vi "TestLV_RT Driver VI.vi"(6 "Device Clock":string) -> ()   [LabVIEW 2017]
uses:
  Par.ctl
  LambdaType.ctl
  Sensor_used.ctl
  <vilib>/Platform/TimedLoop/XDataNode/timing_clust.ctl
  <vilib>/Platform/TimedLoop/XDataNode/nitl_modes.ctl
  <vilib>/Platform/TimedLoop/XDataNode/wakeup.ctl
  <vilib>/SLSC/Initialize Session with Devices.vi
  <vilib>/SLSC/Close Session.vi
  <vilib>/Platform/TimedLoop/XDataNode/XDataNode.xnode
  <vilib>/Platform/TimedLoop/XDataNode/XDNodeRunTimeDep.lvlib
  ALMA_10201-10401_O2SensorSim Engine.lvlib
  <vilib>/SLSC/SLSC.lvlib
  <resource>/objmgr/slsc.rc
panel:
  in  "Feedback 3":string[](array[string])=["Lambda Feedback", "Status", "Duty Cycle Heater", "Frequency Heater", "Ip", "Ri", "V_Ip", "V_Ri"]
  in  "Feedback 2":string[](array[string])=["Lambda Feedback", "Status", "Duty Cycle Heater", "Frequency Heater", "Ip", "Ri", "V_Ip", "V_Ri"]
  in  "Feedback":string[](array[string])=["Lambda Feedback", "Status", "Duty Cycle Heater", "Frequency Heater", "Ip", "Ri", "V_Ip", "V_Ri"]
  in  "Setpoint 2":string[](array[string])=["Enable_1", "Lambda Target_1", "Sensor Temp_1", "Enable_3", "Lambda Target_3", "Sensor Temp_3"]
  in  "Setpoint":string[](array[string])=["Enable_1", "Lambda Target_1", "Sensor Temp_1", "Enable_2", "Lambda Target_2", "Sensor Temp_2", "Enable_3", "Lambda Target_3", "Sensor Temp_3", "Enable_4", "Lambda Target_4", "Sensor Temp_4"]
  in  "Array":T1[](array[typedef])=[0, 1, 2, 3] items=["LSU4.2", "LSU4.9", "LZA03", "LZA08", "Custom", "[mA]"]
  in  "Tab Control":enum32{"Page 1", "Page 2", "Page 3", "Page 4"}(tab)
  out "Temperature [°C] VS Rs [W]":cluster{"Custom Temp":dbl[], "Custom Ohm":dbl[]}(graph)
  out "l VS IP [mA]":T2(graph)
  in  "Mode":enum16{"SLSC Mode", "ANALOG Mode"}(ring)
  out "decimal integer string":string
  out "Dev.ProductName":string
  out "Dev.VendorNum":u32
  out "Dev.ProductNum":u32
  out "output cluster":T3
  out "VS feedback 2":dbl[](array[numeric])=[1.0032000541687012, 0.0, 0.0, 0.0, 1.0032000541687012, 0.0, 99.0, 0.0, -2.0, 1000.0, -2.0, 1000.0, 0.0, 0.0, 3.333400011062622, 9.309800148010254, 3.333400011062622, 9.309800148010254]
  in  "VS control 2":dbl[](array[numeric])=[0.0, 0.0, 0.0, 0.0, 0.0, 0.0, 0.0, 0.0, 0.0, 0.0, 0.0, 0.0, 0.0, 0.0, 0.0]
  in  "#ch_choise":enum16{"O2Sim_2ch", "O2Sim_4ch"}(ring)
  in  "SensorUsed 2":T3
  in  "Next_IP 1":u32=192 caption="O2SensorSim IP"
  in  "Next_IP 4":u32=4
  in  "Next_IP 2":u32=168
  in  "Next_IP 3":u32=1
  out "error out 2":errorcluster
  out "error out":errorcluster
  out "VS feedback":dbl[](array[numeric])
  in  "stop":bool
  in  "VS control":dbl[](array[numeric])=[0.0, 0.0, 0.0, 0.0, 0.0, 0.0, 0.0, 0.0, 0.0, 0.0, 0.0, 0.0, 0.0, 0.0, 0.0, 0.0, 0.0, 0.0, 0.0, 0.0, 0.0]
  in  "devices":refnum<k21>="SLSC-12001-0310EC4F-Mod1"
  in  "par":T4={"Loop time"={"Loop Rate"=0, "Processor"=0}, "COM"={"COM IP"="0.0.0.0", "COM port"=1, "Local port"=0, "Next_IP 1"=0, "Next_IP 2"=0, "Next_IP 3"=0, "Next_IP 4"=0}, "O2Sensor1"={"Lambda"={"LSU4.2 Lambda"=[], "LSU4.2 Ip"=[], "LSU4.9 Lambda"=[], "LSU4.9 Ip"=[], "LZA03 Lambda"=[], "LZA03 Ip"=[], "LZA08 Lambda"=[], "LZA08 Ip"=[], "Custom Lambda"=[], "Custom Ip"=[]}, "Temp"={"LSU4.2 Temp"=[], "LSU4.2 Ohm"=[], "LSU4.9 Temp"=[], "LSU4.9 Ohm"=[], "LZA03 Temp"=[], "LZA03 Ohm"=[], "LZA08 Temp"=[], "LZA08 Ohm"=[], "Custom Temp"=[], "Custom Ohm"=[]}, "Lambda Type"=0, "PID"={"Ki"=0.0, "Kp"=0.0, "Kd"=0.0, "FeedFW"=0.0}}, "O2Sensor2"={"Lambda"={"LSU4.2 Lambda"=[], "LSU4.2 Ip"=[], "LSU4.9 Lambda"=[], "LSU4.9 Ip"=[], "LZA03 Lambda"=[], "LZA03 Ip"=[], "LZA08 Lambda"=[], "LZA08 Ip"=[], "Custom Lambda"=[], "Custom Ip"=[]}, "Temp"={"LSU4.2 Temp"=[], "LSU4.2 Ohm"=[], "LSU4.9 Temp"=[], "LSU4.9 Ohm"=[], "LZA03 Temp"=[], "LZA03 Ohm"=[], "LZA08 Temp"=[], "LZA08 Ohm"=[], "Custom Temp"=[], "Custom Ohm"=[]}, "Lambda Type"=0, "PID"={"Ki"=0.0, "Kp"=0.0, "Kd"=0.0, "FeedFW"=0.0}}, "O2Sensor3"={"Lambda"={"LSU4.2 Lambda"=[], "LSU4.2 Ip"=[], "LSU4.9 Lambda"=[], "LSU4.9 Ip"=[], "LZA03 Lambda"=[], "LZA03 Ip"=[], "LZA08 Lambda"=[], "LZA08 Ip"=[], "Custom Lambda"=[], "Custom Ip"=[]}, "Temp"={"LSU4.2 Temp"=[], "LSU4.2 Ohm"=[], "LSU4.9 Temp"=[], "LSU4.9 Ohm"=[], "LZA03 Temp"=[], "LZA03 Ohm"=[], "LZA08 Temp"=[], "LZA08 Ohm"=[], "Custom Temp"=[], "Custom Ohm"=[]}, "Lambda Type"=0, "PID"={"Ki"=0.0, "Kp"=0.0, "Kd"=0.0, "FeedFW"=0.0}}, "O2Sensor4"={"Lambda"={"LSU4.2 Lambda"=[], "LSU4.2 Ip"=[], "LSU4.9 Lambda"=[], "LSU4.9 Ip"=[], "LZA03 Lambda"=[], "LZA03 Ip"=[], "LZA08 Lambda"=[], "LZA08 Ip"=[], "Custom Lambda"=[], "Custom Ip"=[]}, "Temp"={"LSU4.2 Temp"=[], "LSU4.2 Ohm"=[], "LSU4.9 Temp"=[], "LSU4.9 Ohm"=[], "LZA03 Temp"=[], "LZA03 Ohm"=[], "LZA08 Temp"=[], "LZA08 Ohm"=[], "Custom Temp"=[], "Custom Ohm"=[]}, "Lambda Type"=0, "PID"={"Ki"=0.0, "Kp"=0.0, "Kd"=0.0, "FeedFW"=0.0}}, "Board"=0, "Mode"=enum."SLSC Mode", "vendor.Num"=4141, "product.Num"=0} {"Board" items=["O2Sim_2ch", "O2Sim_4ch"]; "O2Sensor4"."Lambda Type" items=["LSU4.2", "LSU4.9", "LZA03", "LZA08", "Custom", "[mA]"]; "O2Sensor3"."Lambda Type" items=["LSU4.2", "LSU4.9", "LZA03", "LZA08", "Custom", "[mA]"]; "O2Sensor2"."Lambda Type" items=["LSU4.2", "LSU4.9", "LZA03", "LZA08", "Custom", "[mA]"]; "O2Sensor1"."Lambda Type" items=["LSU4.2", "LSU4.9", "LZA03", "LZA08", "Custom", "[mA]"]}
  out "Device Session":refnum<k21>
  out "COM error":bool
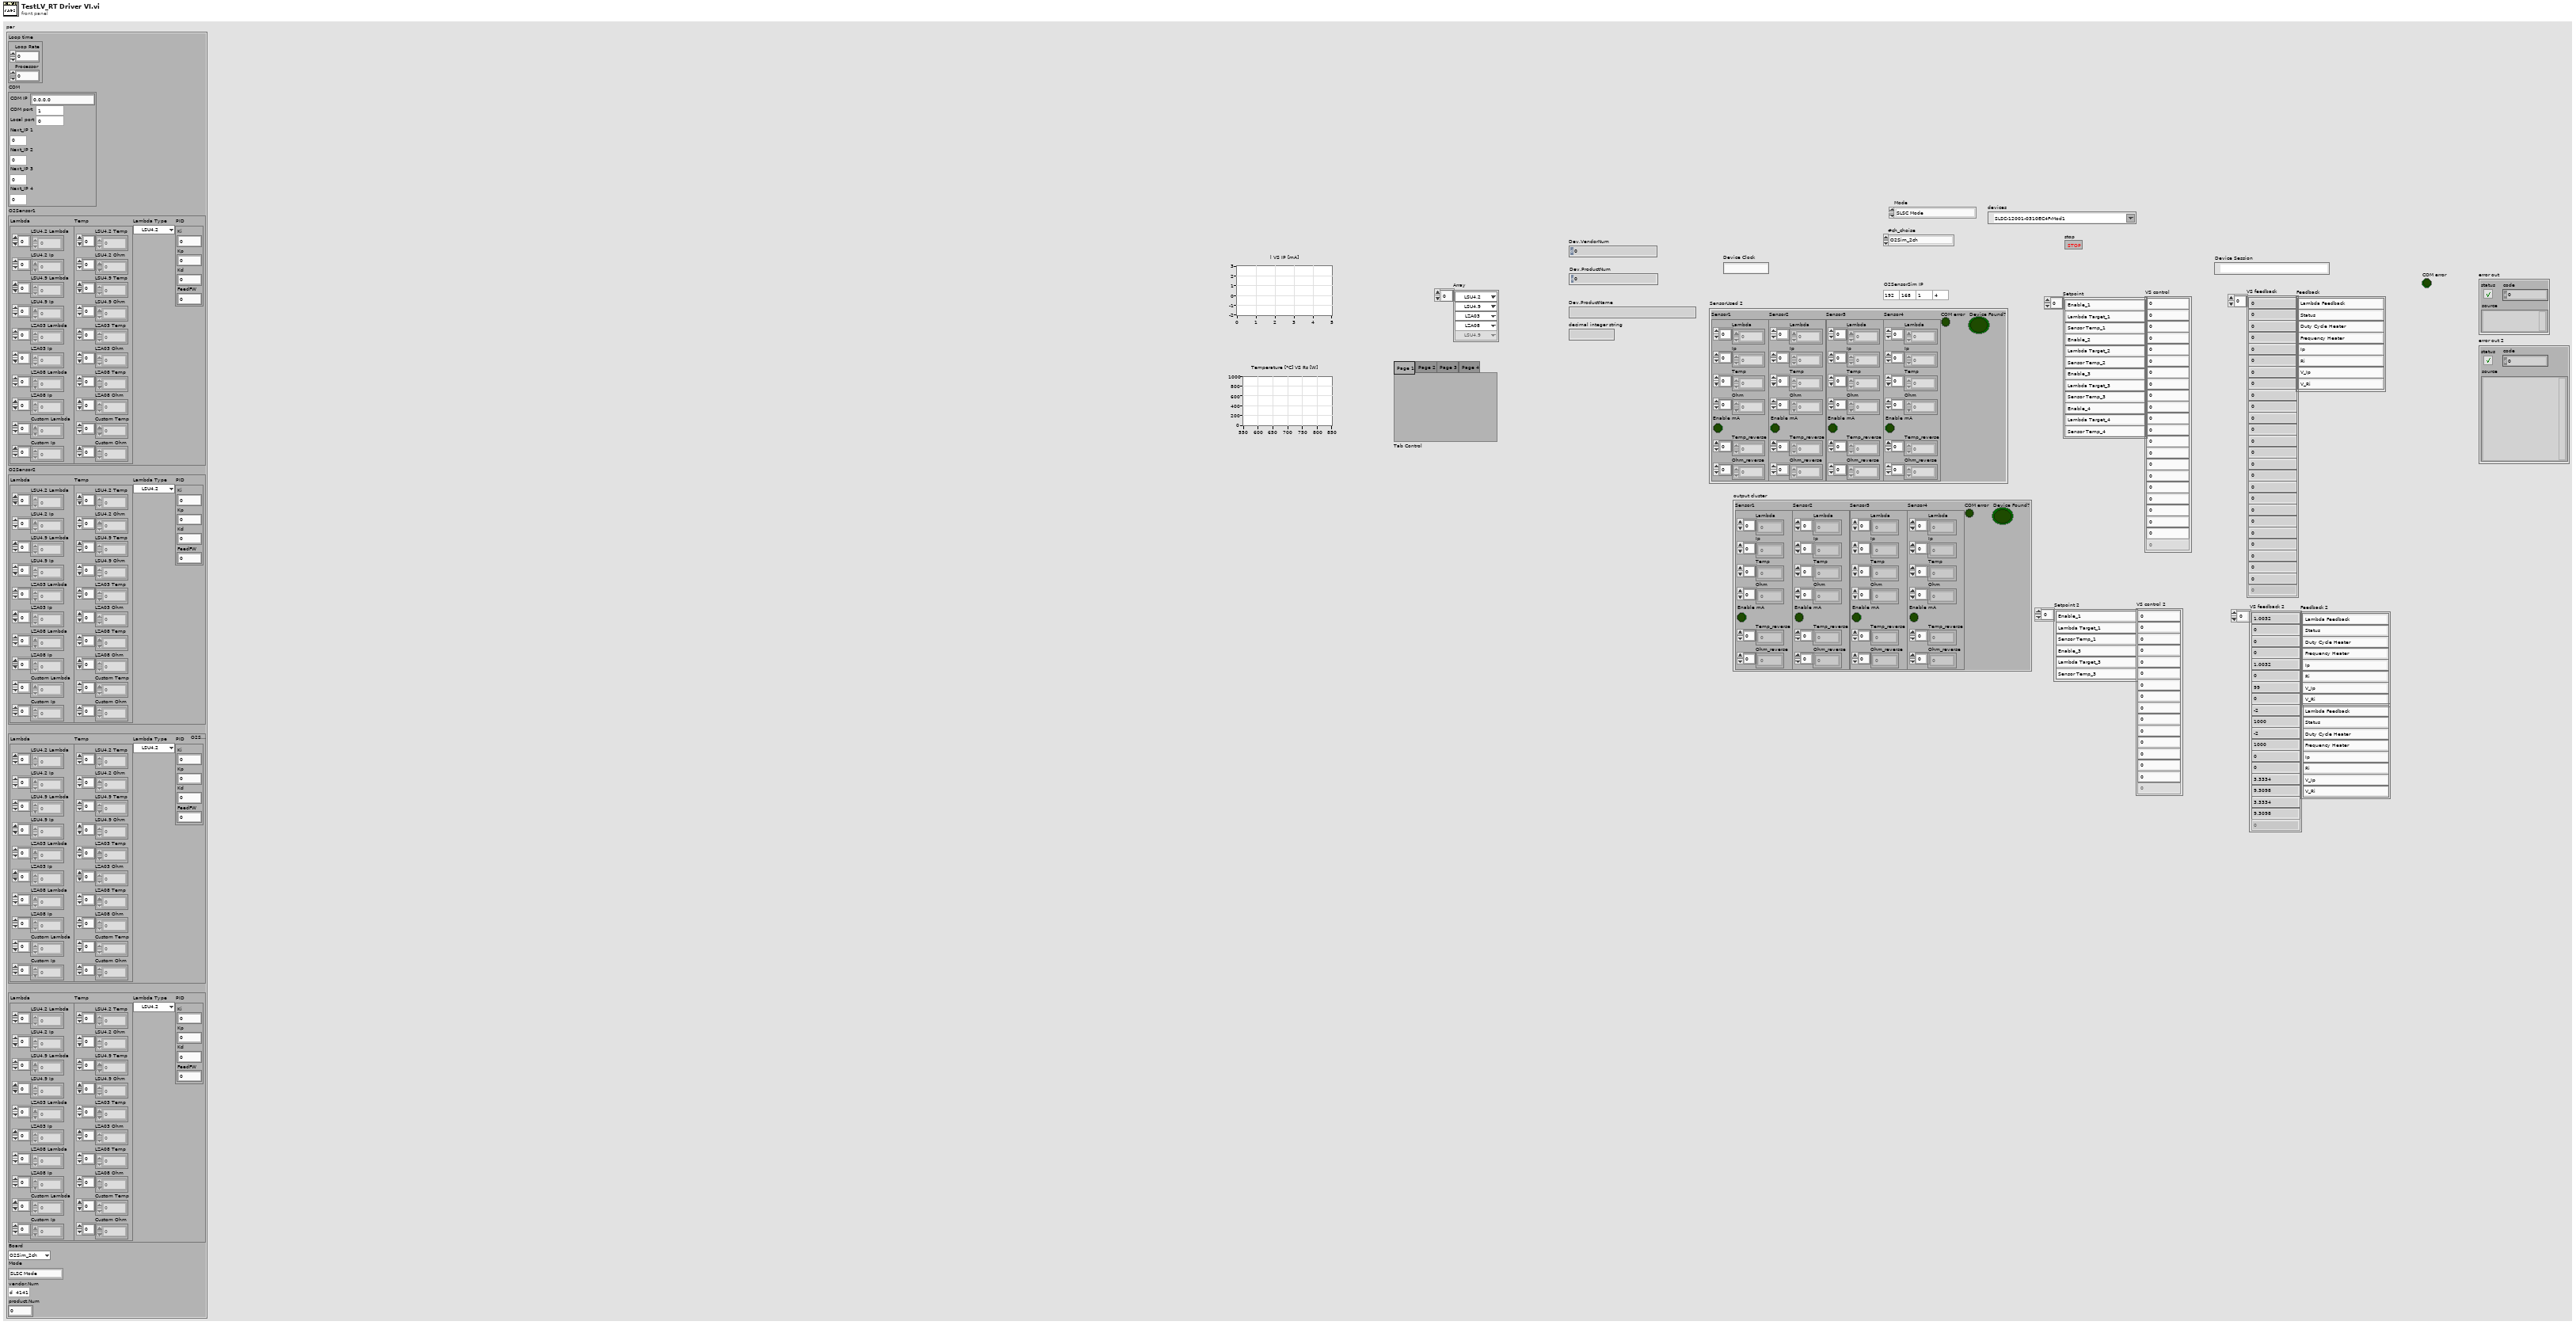
[diagram p1: front panel]
types:
  T1 = typedef "LambdaType.ctl" = u16
  T2 = cluster{"Custom Lambda":dbl[], "Custom Ip":dbl[]}
  T3 = typedef "ALMA_10201-10401_O2SensorSim Engine.lvlib/Sensor_used.ctl" = cluster{"Sensor1":cluster{"Lambda":dbl[], "Ip":dbl[], "Temp":dbl[], "Ohm":dbl[], "Enable mA":bool, "Temp_reverse":dbl[], "Ohm_reverse":dbl[]}, "Sensor2":cluster{"Lambda":dbl[], "Ip":dbl[], "Temp":dbl[], "Ohm":dbl[], "Enable mA":bool, "Temp_reverse":dbl[], "Ohm_reverse":dbl[]}, "Sensor3":cluster{"Lambda":dbl[], "Ip":dbl[], "Temp":dbl[], "Ohm":dbl[], "Enable mA":bool, "Temp_reverse":dbl[], "Ohm_reverse":dbl[]}, "Sensor4":cluster{"Lambda":dbl[], "Ip":dbl[], "Temp":dbl[], "Ohm":dbl[], "Enable mA":bool, "Temp_reverse":dbl[], "Ohm_reverse":dbl[]}, "COM error":bool, "Device Found?":bool}
  T4 = typedef "Par.ctl" = cluster{"Loop time":cluster{"Loop Rate":i64, "Processor":i32}, "COM":cluster{"COM IP":string, "COM port":u64, "Local port":u64, "Next_IP 1":u32, "Next_IP 2":u32, "Next_IP 3":u32, "Next_IP 4":u32}, "O2Sensor1":cluster{"Lambda":cluster{"LSU4.2 Lambda":dbl[], "LSU4.2 Ip":dbl[], "LSU4.9 Lambda":dbl[], "LSU4.9 Ip":dbl[], "LZA03 Lambda":dbl[], "LZA03 Ip":dbl[], "LZA08 Lambda":dbl[], "LZA08 Ip":dbl[], "Custom Lambda":dbl[], "Custom Ip":dbl[]}, "Temp":cluster{"LSU4.2 Temp":dbl[], "LSU4.2 Ohm":dbl[], "LSU4.9 Temp":dbl[], "LSU4.9 Ohm":dbl[], "LZA03 Temp":dbl[], "LZA03 Ohm":dbl[], "LZA08 Temp":dbl[], "LZA08 Ohm":dbl[], "Custom Temp":dbl[], "Custom Ohm":dbl[]}, "Lambda Type":T1, "PID":cluster{"Ki":dbl, "Kp":dbl, "Kd":dbl, "FeedFW":dbl}}, "O2Sensor2":cluster{"Lambda":cluster{"LSU4.2 Lambda":dbl[], "LSU4.2 Ip":dbl[], "LSU4.9 Lambda":dbl[], "LSU4.9 Ip":dbl[], "LZA03 Lambda":dbl[], "LZA03 Ip":dbl[], "LZA08 Lambda":dbl[], "LZA08 Ip":dbl[], "Custom Lambda":dbl[], "Custom Ip":dbl[]}, "Temp":cluster{"LSU4.2 Temp":dbl[], "LSU4.2 Ohm":dbl[], "LSU4.9 Temp":dbl[], "LSU4.9 Ohm":dbl[], "LZA03 Temp":dbl[], "LZA03 Ohm":dbl[], "LZA08 Temp":dbl[], "LZA08 Ohm":dbl[], "Custom Temp":dbl[], "Custom Ohm":dbl[]}, "Lambda Type":T1, "PID":cluster{"Ki":dbl, "Kp":dbl, "Kd":dbl, "FeedFW":dbl}}, "O2Sensor3":cluster{"Lambda":cluster{"LSU4.2 Lambda":dbl[], "LSU4.2 Ip":dbl[], "LSU4.9 Lambda":dbl[], "LSU4.9 Ip":dbl[], "LZA03 Lambda":dbl[], "LZA03 Ip":dbl[], "LZA08 Lambda":dbl[], "LZA08 Ip":dbl[], "Custom Lambda":dbl[], "Custom Ip":dbl[]}, "Temp":cluster{"LSU4.2 Temp":dbl[], "LSU4.2 Ohm":dbl[], "LSU4.9 Temp":dbl[], "LSU4.9 Ohm":dbl[], "LZA03 Temp":dbl[], "LZA03 Ohm":dbl[], "LZA08 Temp":dbl[], "LZA08 Ohm":dbl[], "Custom Temp":dbl[], "Custom Ohm":dbl[]}, "Lambda Type":T1, "PID":cluster{"Ki":dbl, "Kp":dbl, "Kd":dbl, "FeedFW":dbl}}, "O2Sensor4":cluster{"Lambda":cluster{"LSU4.2 Lambda":dbl[], "LSU4.2 Ip":dbl[], "LSU4.9 Lambda":dbl[], "LSU4.9 Ip":dbl[], "LZA03 Lambda":dbl[], "LZA03 Ip":dbl[], "LZA08 Lambda":dbl[], "LZA08 Ip":dbl[], "Custom Lambda":dbl[], "Custom Ip":dbl[]}, "Temp":cluster{"LSU4.2 Temp":dbl[], "LSU4.2 Ohm":dbl[], "LSU4.9 Temp":dbl[], "LSU4.9 Ohm":dbl[], "LZA03 Temp":dbl[], "LZA03 Ohm":dbl[], "LZA08 Temp":dbl[], "LZA08 Ohm":dbl[], "Custom Temp":dbl[], "Custom Ohm":dbl[]}, "Lambda Type":T1, "PID":cluster{"Ki":dbl, "Kp":dbl, "Kd":dbl, "FeedFW":dbl}}, "Board":u16, "Mode":enum16{"SLSC Mode", "ANALOG Mode"}, "vendor.Num":u32, "product.Num":u32}
  T5 = cluster{"Lambda":cluster{"LSU4.2 Lambda":dbl[], "LSU4.2 Ip":dbl[], "LSU4.9 Lambda":dbl[], "LSU4.9 Ip":dbl[], "LZA03 Lambda":dbl[], "LZA03 Ip":dbl[], "LZA08 Lambda":dbl[], "LZA08 Ip":dbl[], "Custom Lambda":dbl[], "Custom Ip":dbl[]}, "Temp":cluster{"LSU4.2 Temp":dbl[], "LSU4.2 Ohm":dbl[], "LSU4.9 Temp":dbl[], "LSU4.9 Ohm":dbl[], "LZA03 Temp":dbl[], "LZA03 Ohm":dbl[], "LZA08 Temp":dbl[], "LZA08 Ohm":dbl[], "Custom Temp":dbl[], "Custom Ohm":dbl[]}, "Lambda Type":T1, "PID":cluster{"Ki":dbl, "Kp":dbl, "Kd":dbl, "FeedFW":dbl}}
  T6 = cluster{"Lambda":cluster{"LSU4.2 Lambda":dbl[], "LSU4.2 Ip":dbl[], "LSU4.9 Lambda":dbl[], "LSU4.9 Ip":dbl[], "LZA03 Lambda":dbl[], "LZA03 Ip":dbl[], "LZA08 Lambda":dbl[], "LZA08 Ip":dbl[], "Custom Lambda":dbl[], "Custom Ip":dbl[]}, "Temp":cluster{"LSU4.2 Temp":dbl[], "LSU4.2 Ohm":dbl[], "LSU4.9 Temp":dbl[], "LSU4.9 Ohm":dbl[], "LZA03 Temp":dbl[], "LZA03 Ohm":dbl[], "LZA08 Temp":dbl[], "LZA08 Ohm":dbl[], "Custom Temp":dbl[], "Custom Ohm":dbl[]}, "Lambda Type":T1, "PID":cluster{"Ki":dbl, "Kp":dbl, "Kd":dbl, "FeedFW":dbl}}[]
  T7 = cluster{"Custom Lambda":dbl[], "Custom Lambda":dbl[], "Custom Lambda":dbl[], "Custom Lambda":dbl[], bool, "Custom Lambda":dbl[], "Custom Lambda":dbl[]}
  T8 = typedef "XDNodeRunTimeDep.lvlib/timing_clust.ctl" = cluster{"Expected End [f-1]":u64, "Actual End [f-1]":u64, "Finished Late? [f-1]":bool, "Expected End [i-1]":u64, "Actual End [i-1]":u64, "Finished Late? [i-1]":bool, "Expected Start [i]":u64, "Actual Start [i]":u64, "Expected Start [f]":u64, "Actual Start [f]":u64, "Source Name":string, "Structure Name":string, "Period":i64, "Deadline":i64, "Offset":i64, "Start":i64, "Priority":i32, "Timeout":i32, "Mode":T9, "Wakeup Reason":T10, "Error":errorcluster, "Source Type":string, "Secondary Source Type":string, "Global End Time":u64, "Global Start Time":u64, "Frame Duration":u64, "Iteration Duration":u64, "Assigned CPU":i32, "I/O Scan Engine Mode":u32}
  T9 = typedef "XDNodeRunTimeDep.lvlib/nitl_modes.ctl" = enum32{"No Change", "Process missed periods, maintain original phase", "Discard missed periods, maintain original phase", "Process missed periods, ignore original phase", "Discard missed periods, ignore original phase"}
  T10 = typedef "XDNodeRunTimeDep.lvlib/wakeup.ctl" = enum32{"Normal", "Aborted", "Asynchronous wakeup", "Timing source error", "Timed loop error", "Timeout"}
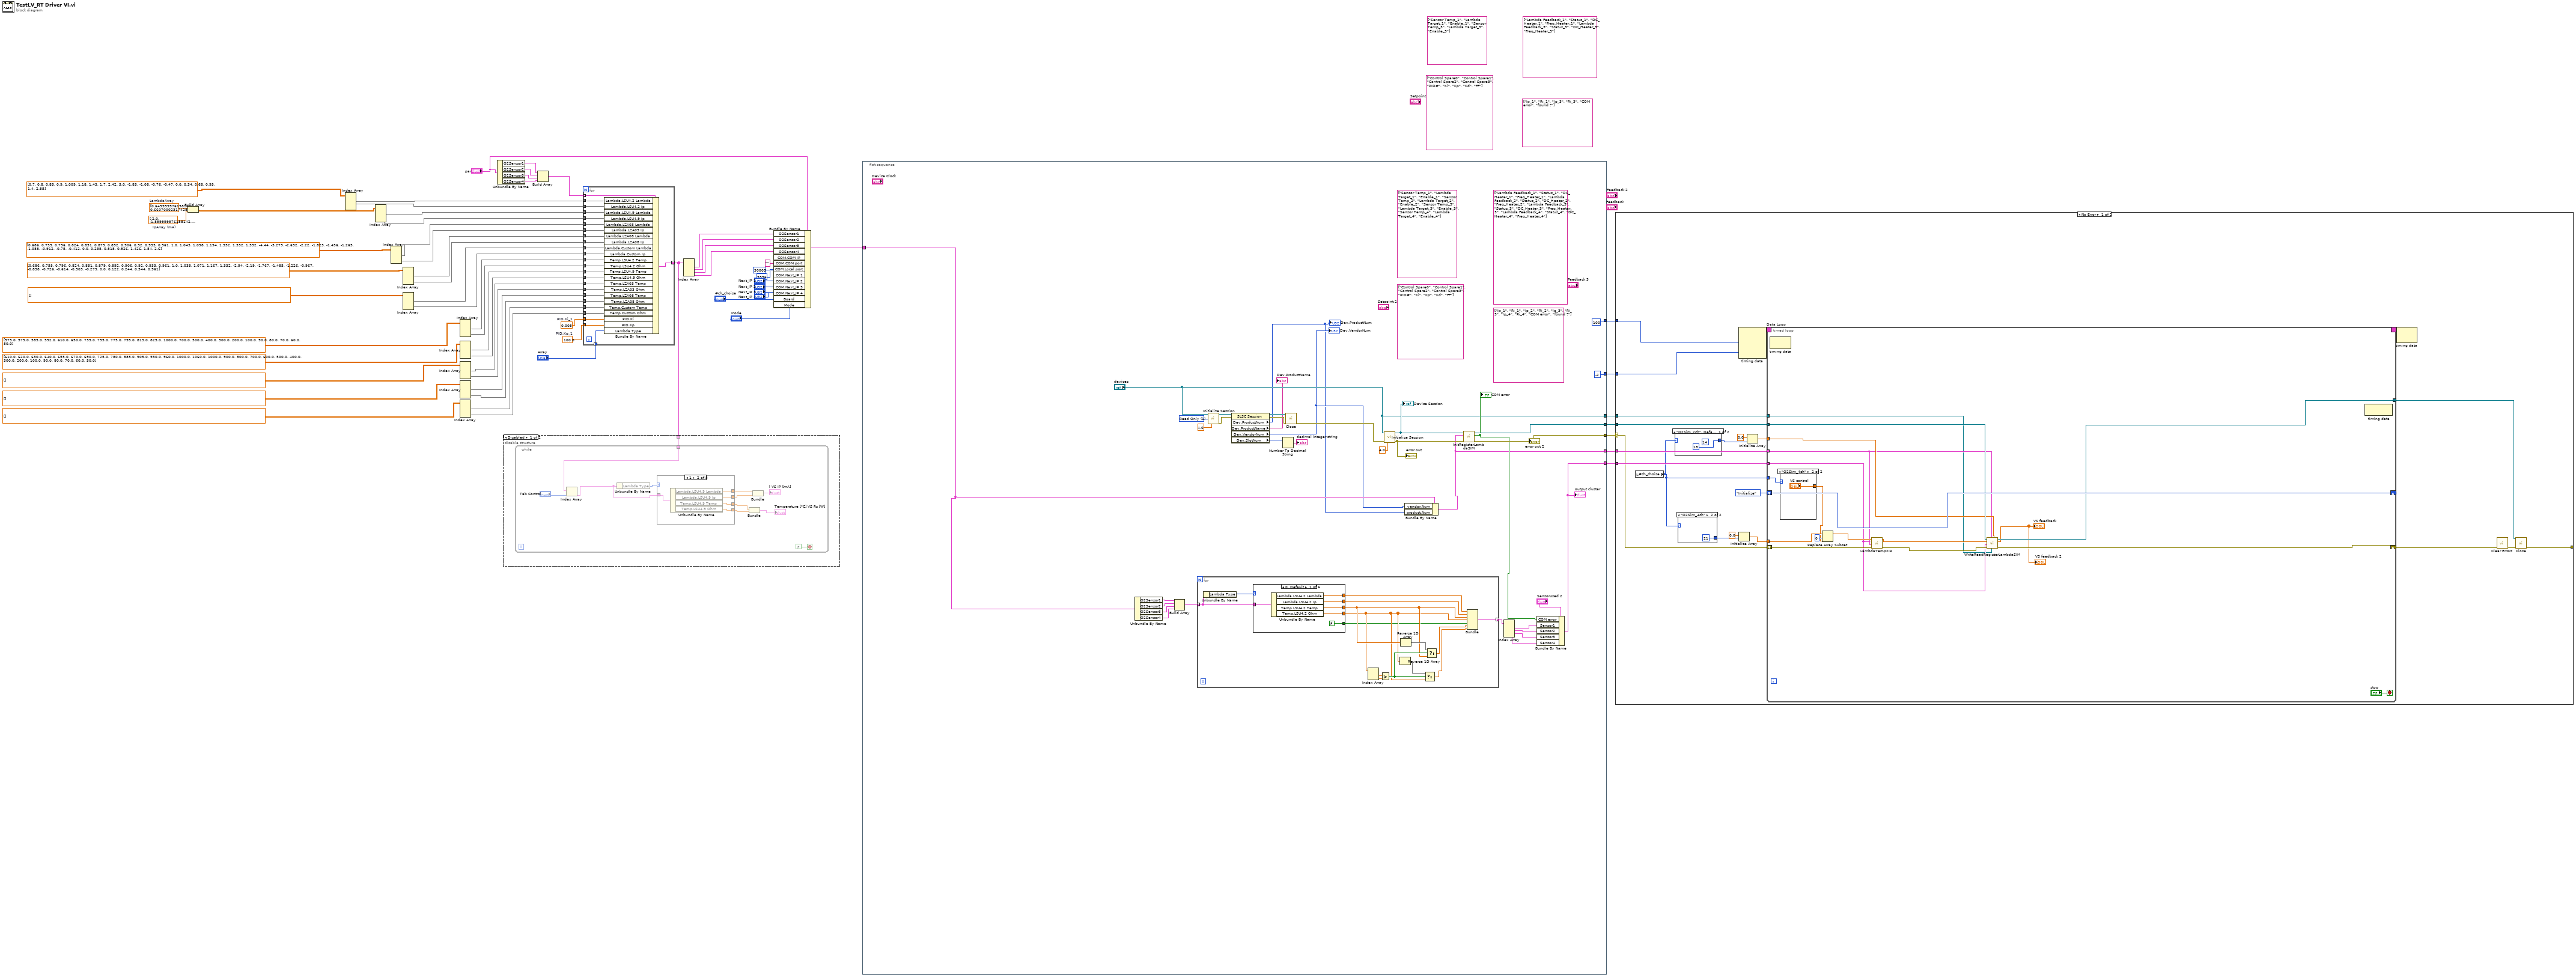
[diagram p0: block diagram]
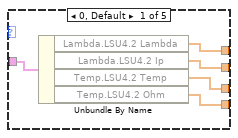
[diagram p2: hidden frame]
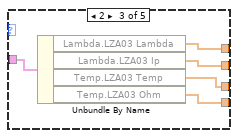
[diagram p3: hidden frame]
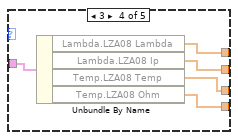
[diagram p4: hidden frame]
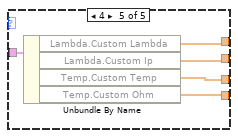
[diagram p5: hidden frame]
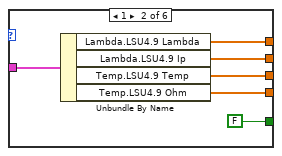
[diagram p7: hidden frame]
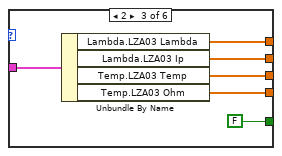
[diagram p8: hidden frame]
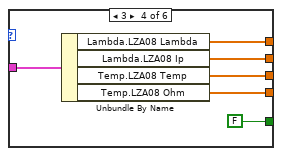
[diagram p9: hidden frame]
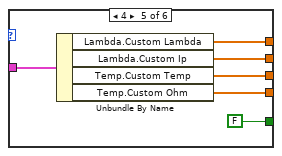
[diagram p10: hidden frame]
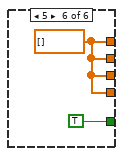
[diagram p11: hidden frame]
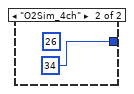
[diagram p12: hidden frame]
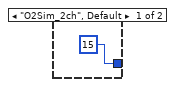
[diagram p13: hidden frame]
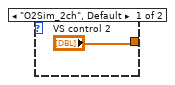
[diagram p14: hidden frame]
diagram:
  (unwired) string[] ["Control Spare0", "Control Spare1", "Control Spare2", "Control Spare3", "PID#", "Ki", "Kp", "Kd", "FF"] ("Additional Control")
  (unwired) string[] ["Ip_1", "Ri_1", "Ip_3", "Ri_3", "COM error", "found ?"] ("O2SensoSim Feedback 3")
  (unwired) string[] ["Lambda Feedback_1", "Status_1", "DC_Heater_1", "Freq_Heater_1", "Lambda Feedback_3", "Status_3", "DC_Heater_3", "Freq_Heater_3"] ("O2SensoSim Feedback 4")
  (unwired) string[] ["Sensor Temp_1", "Lambda Target_1", "Enable_1", "Sensor Temp_3", "Lambda Target_3", "Enable_3"] ("O2SensoSim Setpoint 2")
  w16 = 100.0  # PID.Kp_1
  w17 = 0.005  # PID.Ki_1
  w39 = sgl[] [0.65, 0.6607, 0.6732, 0.6866, 0.7, 0.714, 0.7278, 0.7418, 0.75, 0.7716, 0.7876, 0.7999, 0.8224, 0.841, 0.8502, 0.8802, 0.8999, 0.9501, 0.9791, 0.9895, 1.0, 1.0032, 1.01, 1.0301, 1.0498, 1.077, 1.1, 1.1319, 1.179, 1.1921, 1.2243, 1.2581, 1.3002, 1.331, 1.3703, 1.4289, 1.4554, 1.5016, 1.5504, 1.6021, 1.657, 1.701, 1.7774, 1.8437, 1.9145, 1.9904, 2.0719, 2.1597, 2.2545, 2.3571, 2.4687, 2.5904, 2.7236, 2.8701, 3.0321, 3.212, 3.4131, 3.6393, 3.8958, 4.189, 4.5275, 4.9229, 5.3907, 5.9531, 6.6421, 7.5061, 8.6219, 10.1187, 12.2328, 15.99]  # LambdaArray
  w38 = sgl[] [-2.0, -1.9, -1.8, -1.7, -1.602, -1.5, -1.4, -1.3, -1.243, -1.1, -1.0, -0.927, -0.8, -0.7, -0.652, -0.5, -0.405, -0.183, -0.0746, -0.0398, -0.007, 0.0, 0.0146, 0.057, 0.097, 0.15, 0.193, 0.25, 0.329, 0.35, 0.4, 0.45, 0.509, 0.55, 0.6, 0.67, 0.7, 0.75, 0.8, 0.85, 0.9, 0.938, 1.0, 1.05, 1.1, 1.15, 1.2, 1.25, 1.3, 1.35, 1.4, 1.45, 1.5, 1.55, 1.6, 1.65, 1.7, 1.75, 1.8, 1.85, 1.9, 1.95, 2.0, 2.05, 2.1, 2.15, 2.2, 2.25, 2.3, 2.3565]  # IpArray (mA)
  n1 = Build Array(w39, w38) -> (w37:sgl[][])
  n2 = Index Array(array=dbl[][] [[0.7, 0.8, 0.85, 0.9, 1.009, 1.18, 1.43, 1.7, 2.42, 5.0], [-1.85, -1.08, -0.76, -0.47, 0.0, 0.34, 0.68, 0.95, 1.4, 2.55]] ("appended array 2")) -> (element #1=w36:dbl[], element #2=w55:dbl[])  [unwired: 4 in]
  n3 = Index Array(array=w37) -> (element #1=w57:sgl[], element #2=w56:sgl[])  [unwired: 4 in]
  n4 = Index Array(array=dbl[][] [[0.686, 0.755, 0.796, 0.824, 0.851, 0.879, 0.892, 0.906, 0.92, 0.933, 0.961, 1.0, 1.043, 1.098, 1.194, 1.332, 1.332, 1.332], [-4.44, -3.279, -2.632, -2.22, -1.823, -1.456, -1.265, -1.088, -0.912, -0.75, -0.412, 0.0, 0.235, 0.515, 0.926, 1.426, 1.54, 2.6]] ("appended array")) -> (element #1=w52:dbl[], element #2=w51:dbl[])  [unwired: 4 in]
  n5 = Index Array(array=dbl[][] [[0.686, 0.755, 0.796, 0.824, 0.851, 0.879, 0.892, 0.906, 0.92, 0.933, 0.961, 1.0, 1.035, 1.071, 1.167, 1.332], [-2.94, -2.19, -1.767, -1.485, -1.226, -0.967, -0.838, -0.726, -0.614, -0.503, -0.279, 0.0, 0.122, 0.244, 0.544, 0.961]] ("appended array")) -> (element #1=w50:dbl[], element #2=w49:dbl[])  [unwired: 4 in]
  n6 = Index Array(array=dbl[][] [] ("appended array")) -> (element #1=w48:dbl[], element #2=w47:dbl[])  [unwired: 4 in]
  n7 = Index Array(array=dbl[][] [[575.0, 579.0, 585.0, 592.0, 610.0, 650.0, 735.0, 755.0, 775.0, 795.0, 813.0, 825.0], [1000.0, 700.0, 500.0, 400.0, 300.0, 200.0, 100.0, 90.0, 80.0, 70.0, 60.0, 50.0]] ("appended array")) -> (element #1=w27:dbl[], element #2=w26:dbl[])  [unwired: 4 in]
  n8 = Index Array(array=dbl[][] [[610.0, 620.0, 630.0, 640.0, 655.0, 670.0, 690.0, 725.0, 780.0, 885.0, 905.0, 930.0, 960.0, 1000.0, 1060.0], [1000.0, 900.0, 800.0, 700.0, 600.0, 500.0, 400.0, 300.0, 200.0, 100.0, 90.0, 80.0, 70.0, 60.0, 50.0]] ("appended array")) -> (element #1=w25:dbl[], element #2=w24:dbl[])  [unwired: 4 in]
  n9 = Index Array(array=dbl[][] [] ("appended array")) -> (element #1=w23:dbl[], element #2=w22:dbl[])  [unwired: 4 in]
  n10 = Index Array(array=dbl[][] [] ("appended array")) -> (element #1=w21:dbl[], element #2=w20:dbl[])  [unwired: 4 in]
  n11 = Index Array(array=dbl[][] [] ("appended array")) -> (element #1=w19:dbl[], element #2=w18:dbl[])  [unwired: 4 in]
  n12 = Unbundle By Name("par") -> ("O2Sensor1"=w14:T5, "O2Sensor2"=w33:T5, "O2Sensor3"=w34:T5, "O2Sensor4"=w35:T5)
  n13 = Build Array(w14, w33, w34, w35) -> (w32:T6)
  n14 = for {
    tunnel: w57 -> [w88]
    tunnel: w56 -> [w87]
    tunnel: w55 -> [w86]
    tunnel: w52 -> [w85]
    tunnel: w51 -> [w84]
    tunnel: w50 -> [w83]
    tunnel: w49 -> [w82]
    tunnel: w48 -> [w81]
    tunnel: w47 -> [w80]
    tunnel: w36 -> [w79]
    tunnel: w32 -> [w78] mode=indexing
    tunnel: [w77] -> w2 mode=indexing
    tunnel: w27 -> [w76]
    tunnel: w26 -> [w75]
    tunnel: w25 -> [w74]
    tunnel: w24 -> [w73]
    tunnel: w23 -> [w72]
    tunnel: w22 -> [w71]
    tunnel: w21 -> [w70]
    tunnel: w20 -> [w69]
    tunnel: w19 -> [w68]
    tunnel: w18 -> [w67]
    tunnel: w17 -> [w66]
    tunnel: w16 -> [w65]
    tunnel: "Array" -> [w64] mode=indexing
    n15 = Bundle By Name(cluster=w78, "Lambda.LSU4.2 Lambda"=w79, "Lambda.LSU4.2 Ip"=w86, "Lambda.LSU4.9 Lambda"=w88, "Lambda.LSU4.9 Ip"=w87, "Lambda.LZA03 Lambda"=w85, "Lambda.LZA03 Ip"=w84, "Lambda.LZA08 Lambda"=w83, "Lambda.LZA08 Ip"=w82, "Lambda.Custom Lambda"=w81, "Lambda.Custom Ip"=w80, "Temp.LSU4.2 Temp"=w76, "Temp.LSU4.2 Ohm"=w75, "Temp.LSU4.9 Temp"=w74, "Temp.LSU4.9 Ohm"=w73, "Temp.LZA03 Temp"=w72, "Temp.LZA03 Ohm"=w71, "Temp.LZA08 Temp"=w70, "Temp.LZA08 Ohm"=w69, "Temp.Custom Temp"=w68, "Temp.Custom Ohm"=w67, "PID.Ki"=w66, "PID.Kp"=w65, "Lambda Type"=w64) -> (w77:T5)
  }
  n16 = disable-structure shown="Disabled" {
    disable-tunnel: w2 -> [w89 _]
    frame Disabled {
      n17 = while {
        tunnel: w89 -> [w97]
        stop <- FALSE stop-if-true
        n18 = Index Array(array=w97, index="Tab Control") -> (element=w95:T5)
        n19 = Unbundle By Name(w95) -> ("Lambda Type"=w96:T1)
        n20 = case shown="1" w96 {
          tunnel: w95 -> [w105 w110 w115 w120 w125]
          tunnel: [w104 w109 w114 w119 w124] -> w94
          tunnel: [w103 w108 w113 w118 w123] -> w93
          tunnel: [w102 w107 w112 w117 w122] -> w92
          tunnel: [w101 w106 w111 w116 w121] -> w91
          frame 0, Default {
            n21 = Unbundle By Name(w105) -> ("Lambda.LSU4.2 Lambda"=w104:dbl[], "Lambda.LSU4.2 Ip"=w103:dbl[], "Temp.LSU4.2 Temp"=w102:dbl[], "Temp.LSU4.2 Ohm"=w101:dbl[])
          }
          frame 1 {
            n22 = Unbundle By Name(w110) -> ("Lambda.LSU4.9 Lambda"=w109:dbl[], "Lambda.LSU4.9 Ip"=w108:dbl[], "Temp.LSU4.9 Temp"=w107:dbl[], "Temp.LSU4.9 Ohm"=w106:dbl[])
          }
          frame 2 {
            n23 = Unbundle By Name(w115) -> ("Lambda.LZA03 Lambda"=w114:dbl[], "Lambda.LZA03 Ip"=w113:dbl[], "Temp.LZA03 Temp"=w112:dbl[], "Temp.LZA03 Ohm"=w111:dbl[])
          }
          frame 3 {
            n24 = Unbundle By Name(w120) -> ("Lambda.LZA08 Lambda"=w119:dbl[], "Lambda.LZA08 Ip"=w118:dbl[], "Temp.LZA08 Temp"=w117:dbl[], "Temp.LZA08 Ohm"=w116:dbl[])
          }
          frame 4 {
            n25 = Unbundle By Name(w125) -> ("Lambda.Custom Lambda"=w124:dbl[], "Lambda.Custom Ip"=w123:dbl[], "Temp.Custom Temp"=w122:dbl[], "Temp.Custom Ohm"=w121:dbl[])
          }
        }
        n26 = Bundle("Custom Temp"=w92, "Custom Ohm"=w91) -> (→"Temperature [°C] VS Rs [W]":cluster{"Custom Temp":dbl[], "Custom Ohm":dbl[]})  [unwired: 1 in]
        n27 = Bundle("Custom Lambda"=w94, "Custom Ip"=w93) -> (→"l VS IP [mA]":T2)  [unwired: 1 in]
      }
    }
    frame Enabled {
    }
  }
  n28 = Index Array(array=w2) -> (element #1=w28:T5, element #2=w29:T5, element #3=w30:T5, element #4=w31:T5)  [unwired: 4 in]
  n29 = Bundle By Name(cluster="par", "O2Sensor1"=w28, "O2Sensor2"=w29, "O2Sensor3"=w30, "O2Sensor4"=w31, "COM.COM IP"="", "COM.COM port"=u64 30005 ("Local port"), "COM.Local port"=u64 5556 ("Lambda port"), "COM.Next_IP 1"="Next_IP 1", "COM.Next_IP 2"="Next_IP 2", "COM.Next_IP 3"="Next_IP 3", "COM.Next_IP 4"="Next_IP 4", "Board"="#ch_choise", "Mode"="Mode") -> (w13:T4)
  n30 = flat-sequence {
    tunnel: [i64 100 ("Loop time.Period [ms]")] -> w63
    tunnel: [-2 ("Loop time.Processor")] -> w62
    tunnel: [w160] -> w61
    tunnel: [w159] -> w60
    tunnel: [w126] -> w59
    tunnel: [w130] -> w58
    tunnel: w13 -> [w129]
    tunnel: ["devices"] -> w4
    frame #0 {
      w138 = 1 items=["None"=0, "Read Only"=1, "Read/Write"=3] ("reservation access (Read/Write)")
      (unwired) string[] ["Control Spare0", "Control Spare1", "Control Spare2", "Control Spare3", "PID#", "Ki", "Kp", "Kd", "FF"] ("Additional Control")
      (unwired) string[] ["Ip_1", "Ri_1", "Ip_2", "Ri_2", "Ip_3", "Ri_3", "Ip_4", "Ri_4", "COM error", "found ?"] ("O2SensoSim Feedback 3")
      (unwired) string[] ["Lambda Feedback_1", "Status_1", "DC_Heater_1", "Freq_Heater_1", "Lambda Feedback_2", "Status_2", "DC_Heater_2", "Freq_Heater_2", "Lambda Feedback_3", "Status_3", "DC_Heater_3", "Freq_Heater_3", "Lambda Feedback_4", "Status_4", "DC_Heater_4", "Freq_Heater_4"] ("O2SensoSim Feedback 4")
      (unwired) string[] ["Sensor Temp_1", "Lambda Target_1", "Enable_1", "Sensor Temp_2", "Lambda Target_2", "Enable_2", "Sensor Temp_3", "Lambda Target_3", "Enable_3", "Sensor Temp_4", "Lambda Target_4", "Enable_4"] ("O2SensoSim Setpoint 2")
      n31 = Unbundle By Name(w129) -> ("O2Sensor1"=w157:T5, "O2Sensor2"=w156:T5, "O2Sensor3"=w155:T5, "O2Sensor4"=w154:T5)
      n32 = Build Array(w157, w156, w155, w154) -> (w153:T6)
      n33 = for {
        tunnel: w153 -> [w162] mode=indexing
        tunnel: [w163] -> w152 mode=indexing
        n34 = Unbundle By Name(w162) -> ("Lambda Type"=w161:T1)
        n35 = case shown="0, Default" w161 {
          tunnel: w162 -> [w181 w187 w193 w199 w205 _]
          tunnel: [w179 w185 w191 w197 w203 w206] -> w170
          tunnel: [w178 w184 w190 w196 w202 w206] -> w169
          tunnel: [FALSE FALSE FALSE FALSE FALSE TRUE] -> w166
          tunnel: [w177 w183 w189 w195 w201 w206] -> w168
          tunnel: [w176 w182 w188 w194 w200 w206] -> w167
          frame 0, Default {
            n36 = Unbundle By Name(w181) -> ("Lambda.LSU4.2 Lambda"=w179:dbl[], "Lambda.LSU4.2 Ip"=w178:dbl[], "Temp.LSU4.2 Temp"=w177:dbl[], "Temp.LSU4.2 Ohm"=w176:dbl[])
          }
          frame 1 {
            n37 = Unbundle By Name(w187) -> ("Lambda.LSU4.9 Lambda"=w185:dbl[], "Lambda.LSU4.9 Ip"=w184:dbl[], "Temp.LSU4.9 Temp"=w183:dbl[], "Temp.LSU4.9 Ohm"=w182:dbl[])
          }
          frame 2 {
            n38 = Unbundle By Name(w193) -> ("Lambda.LZA03 Lambda"=w191:dbl[], "Lambda.LZA03 Ip"=w190:dbl[], "Temp.LZA03 Temp"=w189:dbl[], "Temp.LZA03 Ohm"=w188:dbl[])
          }
          frame 3 {
            n39 = Unbundle By Name(w199) -> ("Lambda.LZA08 Lambda"=w197:dbl[], "Lambda.LZA08 Ip"=w196:dbl[], "Temp.LZA08 Temp"=w195:dbl[], "Temp.LZA08 Ohm"=w194:dbl[])
          }
          frame 4 {
            n40 = Unbundle By Name(w205) -> ("Lambda.Custom Lambda"=w203:dbl[], "Lambda.Custom Ip"=w202:dbl[], "Temp.Custom Temp"=w201:dbl[], "Temp.Custom Ohm"=w200:dbl[])
          }
          frame 5 {
            w206 = dbl[] [] ("Custom Lambda")
          }
        }
        n41 = Index Array(array=w167) -> (element #1=w173:dbl, element #2=w174:dbl)  [unwired: 2 in]
        n42 = Greater?(x=w173, y=w174) -> (0:w171:bool)
        n43 = Reverse 1D Array(array=w167) -> (reversed array=w175:dbl[])
        n44 = Reverse 1D Array(array=w168) -> (reversed array=w172:dbl[])
        n45 = Select(t=w175, s=w171, f=w167) -> (s? t:f=w164:dbl[])
        n46 = Select(t=w172, s=w171, f=w168) -> (s? t:f=w165:dbl[])
        n47 = Bundle("Custom Lambda"=w170, "Custom Lambda"=w169, "Custom Lambda"=w168, "Custom Lambda"=w167, w166, "Custom Lambda"=w165, "Custom Lambda"=w164) -> (w163:T7)  [unwired: 1 in]
      }
      n48 = call-poly <vilib>:"Initialize Session.vi"("devices"="devices", "reservation access (Read/Write)"=w138, "connect timeout (60 sec)"=4.0) -> ("session out"=w142:refnum<k21>, "error out"=w141:errorcluster)  [unwired: 11 in]
      n49 = property class="SLSC Session"(reference=w142, error in=w141) -> (reference out=w140:refnum<k21>, error out=w139:errorcluster, "Dev.ProductNum"=w127:u32, "Dev.ProductName"=→"Dev.ProductName":string, "Dev.VendorNum"=w128:u32, "Dev.SlotNum"=w137:u32)
      "Dev.ProductNum" <- w127
      "Dev.VendorNum" <- w128
      n50 = Number To Decimal String(number=w137) -> (decimal integer string=→"decimal integer string":string)  [unwired: 1 in]
      n51 = call-poly <vilib>:"Close.vi"("session in"=w140, "error in (no error)"=w139) -> ("error out"=w135:errorcluster)  [unwired: 13 in]
      n52 = call-poly <vilib>:"Initialize Session.vi"("devices"="devices", "error in (no error)"=w135, "connect timeout (60 sec)"=4.0) -> ("session out"=w146:refnum<k21>, "error out"=w145:errorcluster)  [unwired: 11 in]
      "Device Session" <- w146
      "error out" <- w145
      n53 = Bundle By Name(cluster=w129, "vendor.Num"=w128, "product.Num"=w127) -> (w126:T4)
      n54 = call "InitRegisterLambdaSIM.vi"("error in"=w145, "value"=w126, "session in"=w146) -> ("error out"=w160:errorcluster, "COM error"=w143:bool, "session out"=w159:refnum<k21>)  [unwired: 6 in]
      "COM error" <- w143
      "error out 2" <- w160
      n55 = Index Array(array=w152) -> (element #1=w131:T7, element #2=w151:T7, element #3=w150:T7, element #4=w149:T7)  [unwired: 4 in]
      n56 = Bundle By Name(cluster="SensorUsed 2", "COM error"=w143, "Sensor1"=w131, "Sensor2"=w151, "Sensor3"=w150, "Sensor4"=w149) -> (w130:T3)
      "output cluster" <- w130
    }
  }
  n57 = case shown="No Error" w61 {
    selector: w61 -> [w212 w260]
    tunnel: [w217 w260] -> _
    tunnel: w63 -> [w224 _]
    tunnel: w62 -> [w223 _]
    tunnel: w59 -> [w221 _]
    tunnel: w60 -> [w220 _]
    tunnel: w58 -> [w218 _]
    tunnel: w4 -> [w209 _]
    frame No Error {
      n58 = local read "#ch_choise"() -> (w208:enum16{"O2Sim_2ch", "O2Sim_4ch"})
      n59 = case shown="\"O2Sim_2ch\", Default" w208 {
        tunnel: [18 ("dimension size") 34 ("dimension size")] -> w214
        frame "O2Sim_2ch", Default {
          (unwired) 14 ("dimension size")
        }
        frame "O2Sim_4ch" {
          (unwired) 26 ("dimension size")
        }
      }
      n60 = case shown="\"O2Sim_4ch\"" w208 {
        tunnel: [15 ("dimension size") 21 ("dimension size")] -> w213
        frame "O2Sim_2ch", Default {
        }
        frame "O2Sim_4ch" {
        }
      }
      n61 = node-c288(w224, w223) -> (w226:T8)  [unwired: 2 in]
      n62 = Initialize Array(0.0 ("element"), w213) -> (w227:dbl[])
      n63 = Initialize Array(0.0 ("element"), w214) -> (w215:dbl[])
      n64 = timed-loop "Data Loop" {
        shift-right: [w235] -> w210
        shift-left: w212 -> [w250]
        timing: w226 -> [_]
        timing-out: [_] -> w225
        shift-right: [w248] -> _
        shift-left: enum16{"Initialize", "Send", "Idle", "Exit"}."Initialize" ("Command") -> [w248]
        tunnel: w221 -> [w238]
        tunnel: w220 -> [w247]
        tunnel: [w246] -> w219
        tunnel: w218 -> [w237]
        tunnel: w227 -> [w249]
        tunnel: w215 -> [w239]
        tunnel: w209 -> [w236]
        tunnel: w208 -> [w233]
        stop <- "stop" stop-if-true
        n65 = node-c288() -> ()  [unwired: 1 in, 1 out]
        n66 = case shown="\"O2Sim_4ch\"" w233 {
          tunnel: ["VS control 2" "VS control"] -> w241
          frame "O2Sim_2ch", Default {
          }
          frame "O2Sim_4ch" {
          }
        }
        n67 = Replace Array Subset(array=w249, new element=w241, index=0) -> (w245:dbl[])
        n68 = call "LambdaTemp2IR.vi"("error constant"=w250, "par 3"=w238, "SensorUsed"=w237, "VS control"=w245) -> ("error constant out"=w243:errorcluster, "VS control out"=w244:dbl[])  [unwired: 6 in]
        n69 = call "WriteReadRegisterLambdaSIM.vi"("VS feedback"=w239, "devices 2"=w236, "par 3"=w238, "error in"=w243, "SensorUsed"=w237, "VS Control"=w244, "session in"=w247) -> ("error out"=w235:errorcluster, "VS feedback"=→"VS feedback" →"VS feedback 2":dbl[], "session out"=w246:refnum<k21>)  [unwired: 2 in]
        n70 = node-c288() -> ()  [unwired: 1 in, 1 out]
      }
      n71 = node-c288(w225) -> ()  [unwired: 1 out]
      n72 = call <vilib>:"Clear Errors.vi"("error in (no error)"=w210) -> ("error out"=w211:errorcluster)  [unwired: 5 in, 1 out]
      n73 = call-poly <vilib>:"Close.vi"("session in"=w219, "error in (no error)"=w211) -> ("error out"=w217:errorcluster)  [unwired: 13 in]
    }
    frame Error {
    }
  }
